vi "End Cube to Corridor.vi"(8 "Command Info In":T1, 10 "End Cube-->Corridor":T5, 11 "Starting Position":T4) -> (0 "Command Info Out":T1)   [LabVIEW 2017]
uses:
  Block Clusters/End Cube--Corridor.ctl
  <vilib>/Rock Robotics/WPI/Framework/Command Status Info.ctl
  <vilib>/Rock Robotics/WPI/Framework/Completion Status.ctl
  <vilib>/Rock Robotics/WPI/Framework/Completion Notifier.ctl
  Support Code/Starting Position.ctl
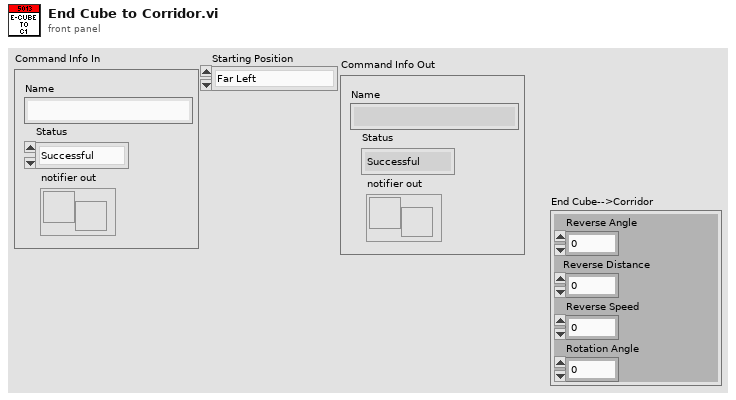
[diagram p1: front panel]
types:
  T1 = typedef "Command Status Info.ctl" = cluster{"Name":string, "Status":T2, "notifier out":T3}
  T2 = typedef "Completion Status.ctl" = enum16{"Successful", "Aborted", "Incomplete"}
  T3 = typedef "Completion Notifier.ctl" = refnum<notifier>
  T4 = typedef "Starting Position.ctl" = enum16{"Far Left", "Center", "Far Right"}
  T5 = typedef "End Cube--Corridor.ctl" = cluster{"Reverse Angle":dbl, "Reverse Distance":dbl, "Reverse Speed ":dbl, "Rotation Angle ":dbl}
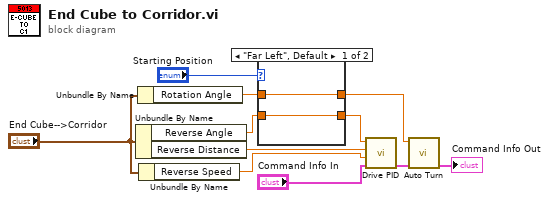
[diagram p0: block diagram]
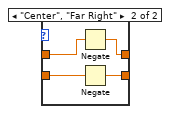
[diagram p2: hidden frame]
diagram:
  n1 = Unbundle By Name("End Cube-->Corridor") -> ("Reverse Angle"=w5:dbl, "Reverse Distance"=w9:dbl)
  n2 = Unbundle By Name("End Cube-->Corridor") -> ("Rotation Angle"=w2:dbl)
  n3 = Unbundle By Name("End Cube-->Corridor") -> ("Reverse Speed"=w8:dbl)
  n4 = case shown="\"Far Left\", Default" "Starting Position" {
    tunnel: w5 -> [w12 w17]
    tunnel: [w12 w14] -> w4
    tunnel: [w13 w15] -> w3
    tunnel: w2 -> [w13 w16]
    frame "Far Left", Default {
    }
    frame "Center", "Far Right" {
      n5 = Negate(x=w16) -> (-x=w15:dbl)
      n6 = Negate(x=w17) -> (-x=w14:dbl)
    }
  }
  n7 = call "Drive PID.vi"("Command Info In"="Command Info In", "Speed"=w8, "Distance"=w9, "Target Angle"=w4) -> ("Command Info Out"=w11:T1)  [unwired: 7 in]
  n8 = call "Auto Turn.vi"("Command Info In"=w11, "Target Angle"=w3) -> ("Command Info Out"=→"Command Info Out":T1)  [unwired: 9 in]
